vi "ArmGetSetpointValue.vi"(8 "ArmSetpoints":T1) -> (0 "Setpoint":dbl)   [LabVIEW 2023]
doc: "Gets arm position depending enum value"
uses:
  ArmGetSetpointEnum.ctl
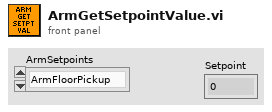
[diagram p1: front panel]
types:
  T1 = typedef "ArmGetSetpointEnum.ctl" = enum16{"ArmFloorPickup", "ArmAmpDeposit", "ArmSpeakerShoot", "ArmStartPosition", "ArmRestPosition", "ArmSourceIntake", "ArmAwayShoot"}
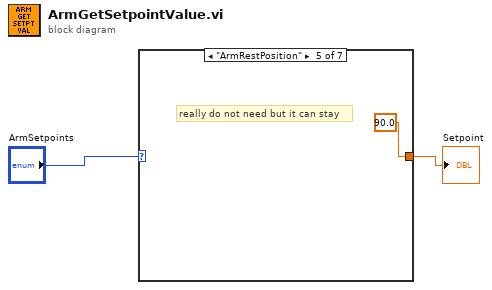
[diagram p0: block diagram]
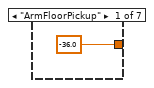
[diagram p2: hidden frame]
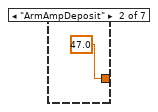
[diagram p3: hidden frame]
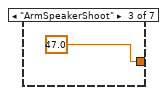
[diagram p4: hidden frame]
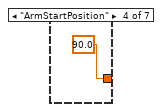
[diagram p5: hidden frame]
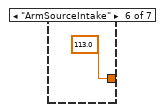
[diagram p6: hidden frame]
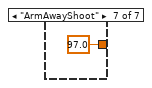
[diagram p7: hidden frame]
diagram:
  n1 = case shown="\"ArmRestPosition\"" "ArmSetpoints" {
    tunnel: [-36.0 ("y") 47.0 ("y") 47.0 ("y") 90.0 ("y") 90.0 ("y") 113.0 ("y") 97.0 ("y")] -> w1
    frame "ArmFloorPickup" {
    }
    frame "ArmAmpDeposit" {
    }
    frame "ArmSpeakerShoot" {
    }
    frame "ArmStartPosition" {
    }
    frame "ArmRestPosition" {
      # "really do not need but it can stay"
    }
    frame "ArmSourceIntake" {
    }
    frame "ArmAwayShoot" {
    }
  }
  "Setpoint" <- w1
